vi "getDelayClusterNames.vi"(1 "appended array":refnum<vi>[](array[refnum])) -> (0 "spreadsheet string":string)   [LabVIEW 2020]
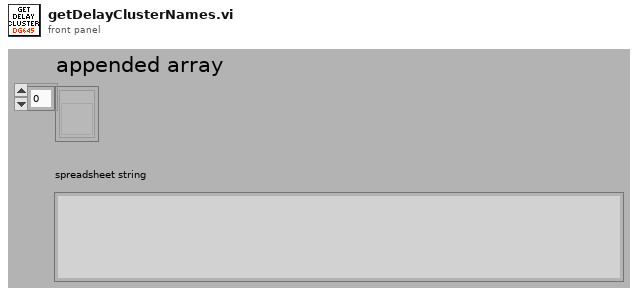
[diagram p1: front panel]
types:
  T1 = typedef "DelayControl_For Multiple Channels.ctl" = cluster{"Channel":string, "Linked":T2, "Delay":T3}
  T2 = typedef "channels_TypDef.ctl" = enum16{"T0", "T1", "A", "B", "C", "D", "E", "F", "G", "H"}
  T3 = typedef "DelayControl2.ctl" = dbl
  T4 = typedef "Type Descriptor Enumeration__ogtk.ctl" = enum8{"<Null>", "I8", "I16", "I32", "I64", "U8", "U16", "U32", "U64", "SGL", "DBL", "EXT", "CSG", "CDB", "CXT", "0x0F", "0x10", "0x11", "0x12", "0x13", "0x14", "Enum U8", "Enum U16", "Enum U32", "Enum U64", "SGL PQ", "DBL PQ", "EXT PQ", "CSG PQ", "CDB PQ", "CXT PQ", "0x1F", "0x20", "Boolean", "0x22", "0x23", "0x24", "0x25", "0x26", "0x27", "0x28", "0x29", "0x2A", "0x2B", "0x2C", "0x2D", "0x2E", "0x2F", "String", "0x31", "Path", "Pict", "0x34", "0x35", "0x36", "DAQ", "0x38", "0x39", "0x3A", "0x3B", "0x3C", "0x3D", "0x3E", "0x3F", "Array", "0x41", "0x42", "0x43", "0x44", "0x45", "0x46", "0x47", "0x48", "0x49", "0x4A", "0x4B", "0x4C", "0x4D", "0x4E", "0x4F", "Cluster", "0x51", "0x52", "Variant", "Waveform", "0x55", "0x56", "0x57", "0x58", "0x59", "0x5A", "0x5B", "0x5C", "0x5D", "0x5E", "0x5F", "0x60", "0x61", "0x62", "0x63", "0x64", "0x65", "0x66", "0x67", "0x68", "0x69", "0x6A", "0x6B", "0x6C", "0x6D", "0x6E", "0x6F", "Refnum"}
  T5 = enum8{"Enabled", "Disabled", "Disabled and Grayed Out"}
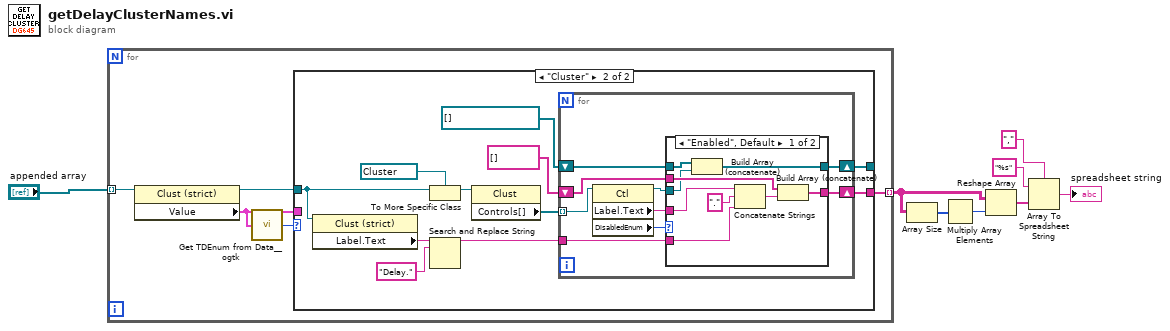
[diagram p0: block diagram]
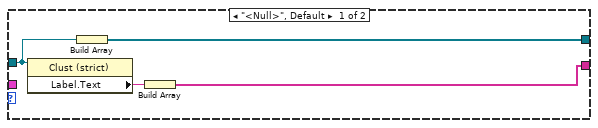
[diagram p2: hidden frame]
diagram:
  n1 = for {
    tunnel: "appended array" -> [w13] mode=indexing
    tunnel: [w9] -> w7 mode=indexing
    n2 = property class="Clust (strict)"(reference=w13) -> (reference out=w10:refnum<vi>, "Value"=w11:T1)  [unwired: 1 in, 1 out]
    n3 = call <userlib>:"Get TDEnum from Data__ogtk.vi"("Data"=w11) -> ("Type Descriptor Enumeration"=w12:T4)  [unwired: 4 in]
    n4 = case shown="\"Cluster\"" w12 {
      tunnel: w11 -> [_ _]
      tunnel: w10 -> [w16 w21]
      tunnel: [w14 w25] -> w9
      tunnel: [w17 w23] -> _
      frame "<Null>", Default {
        n5 = property class="Clust (strict)"(reference=w16) -> ("Label.Text"=w15:string)  [unwired: 1 in, 2 out]
        n6 = Build Array(w16) -> (w17:refnum<vi>[])
        n7 = Build Array(w15) -> (w14:string[])
      }
      frame "Cluster" {
        n8 = property class="Clust (strict)"(reference=w21) -> ("Label.Text"=w20:string)  [unwired: 1 in, 2 out]
        n9 = To More Specific Class(target class=refnum<vi> refnum ("specific class reference"), reference=w21) -> (specific class reference=w27:refnum<vi>)  [unwired: 1 in, 1 out]
        n10 = Search and Replace String(input string=w20, search string="Delay.") -> (result string=w19:string)  [unwired: 6 in, 3 out]
        n11 = property class="Clust"(reference=w27) -> ("Controls[]"=w26:refnum<vi>[])  [unwired: 1 in, 2 out]
        n12 = for {
          tunnel: w26 -> [w37] mode=indexing
          shift-right: [w34] -> w25
          shift-left: string[] [] -> [w36]
          shift-right: [w31] -> w23
          shift-left: refnum<vi>[] [] -> [w30]
          tunnel: w19 -> [w29]
          n13 = property class="Ctl"(reference=w37) -> (reference out=w32:refnum<vi>, "Label.Text"=w35:string, "DisabledEnum"=w33:T5)  [unwired: 1 in, 1 out]
          n14 = case shown="\"Enabled\", Default" w33 {
            tunnel: w36 -> [w45 w48]
            tunnel: w35 -> [w39 _]
            tunnel: [w46 w48] -> w34
            tunnel: w32 -> [w44 _]
            tunnel: [w43 w47] -> w31
            tunnel: w30 -> [w42 w47]
            tunnel: w29 -> [w40 _]
            frame "Enabled", Default {
              n15 = Build Array (concatenate)(w42, w44) -> (w43:refnum<vi>[])
              n16 = Concatenate Strings(w39, "." ("string"), w40) -> (w38:string)
              n17 = Build Array (concatenate)(w45, w38) -> (w46:string[])
            }
            frame "Disabled" {
            }
          }
        }
      }
    }
  }
  n18 = Array Size(array=w7) -> (size(s)=w6:i32[])
  n19 = Multiply Array Elements(1:w6) -> (0:w8:i32)
  n20 = Reshape Array(w7, w8) -> (w3:string[])
  n21 = Array To Spreadsheet String(delimiter (Tab)=",", array=w3, 3:"%s" ("format string")) -> (spreadsheet string=→"spreadsheet string":string)
